vi "Ex4.vi"() -> ()   [LabVIEW 2010]
uses:
  ROS/Code/Slider.ctl
  ROS/Code/JointPositions.ctl
panel:
  in  "Joint Positions":T1 {"left_w2" scale=-180.0..180.0; "left_w1" scale=-180.0..180.0; "left_w0" scale=-180.0..180.0; "left_e1" scale=-180.0..180.0; "left_e0" scale=-180.0..180.0; "left_s1" scale=-180.0..180.0; "left_s0" scale=-180.0..180.0; "right_s1" scale=-180.0..180.0; "right_s0" scale=-180.0..180.0; "right_w2" scale=-180.0..180.0; "right_e1" scale=-180.0..180.0; "right_e0" scale=-180.0..180.0; "right_w0" scale=-180.0..180.0; "right_w1" scale=-180.0..180.0}
  in  "stop":bool
  # "Control Baxter's Arms using the supplied Position Controller"
  # "Currently fails to open /robot/limb/right/command_joint_angles due to issue 2 - Multiple Publishers in Loop \n(https://github.com/chris-smith/ROSforLabview/issues/2)"
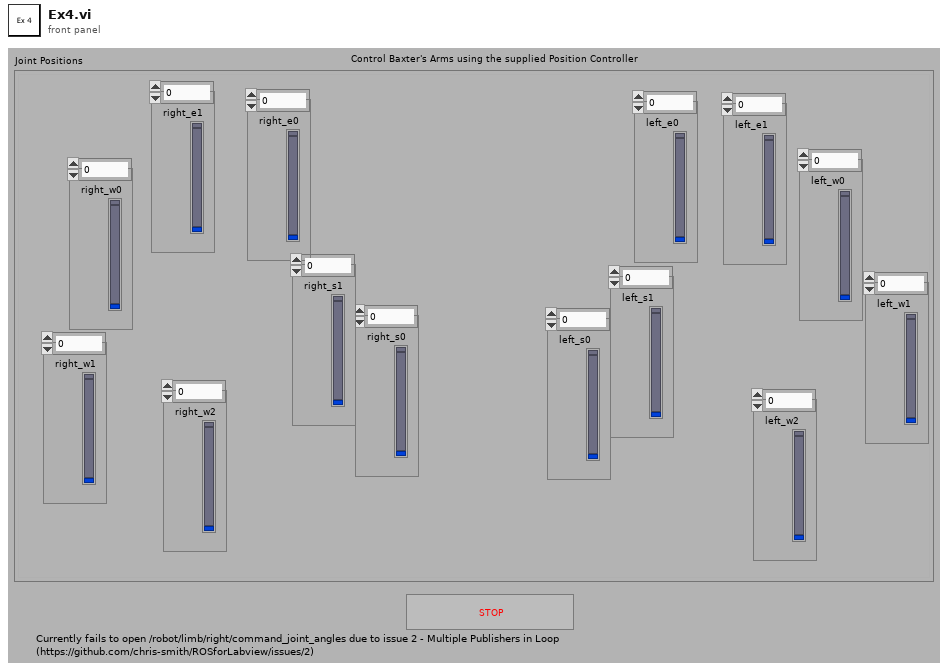
[diagram p1: front panel]
types:
  T1 = typedef "JointPositions.ctl" = cluster{"left_e0":T2, "left_e1":T2, "left_s0":T2, "left_s1":T2, "left_w0":T2, "left_w1":T2, "left_w2":T2, "right_e0":T2, "right_e1":T2, "right_s0":T2, "right_s1":T2, "right_w0":T2, "right_w1":T2, "right_w2":T2}
  T2 = typedef "Slider.ctl" = dbl
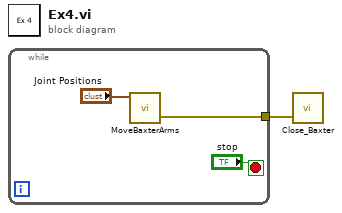
[diagram p0: block diagram]
diagram:
  n1 = while {
    tunnel: [w2] -> w1
    stop <- "stop" stop-if-true
    n2 = call "MoveBaxterArms.vi"("Parameters"="Joint Positions") -> ("error out"=w2:errorcluster)  [unwired: 5 in]
  }
  n3 = call "Close_Baxter.vi"("error in"=w1) -> ()  [unwired: 3 in, 1 out]
